vi "ChoosePass.vi"(8 "error in (no error)":errorcluster, 10 "Game":refnum<class "Game.lvclass">, 11 "Play in":refnum<class "Play.lvclass">) -> (0 "error out":errorcluster, 2 "Receptor passe":enum16{"Striker", "2nd Striker"}(ring), 3 "Play out":refnum<class "Play.lvclass">)   [LabVIEW 2018, in "Play.lvclass"]
uses:
  Play.lvclass
  Game_class/Game.lvclass
  Utilities_class/Utilities.lvclass
  Game_class/Game.lvclass/Game.ctl
  Team_class/Team.lvclass/Team.ctl
  Object_class/Object.lvclass/Object.ctl
  Robot_class/Robot.lvclass/Robot.ctl
  Referee_class/Referee.lvclass/Referee.ctl
  Object_class/Read x.vi
  Object_class/Read y.vi
  Robot_class/Read id.vi
  Referee_class/Read enemy_goalie_id.vi
  Team_class/Read RobotRef.vi
  Game_class/Read AllyRef.vi
  Game_class/Read BallRef.vi
  Game_class/Read FieldRef.vi
  Game_class/Read EnemyRef.vi
  Game_class/Read Referee.vi
  Ball_class/Ball.lvclass
  Ally_class/Ally.lvclass
  Robot_class/Robot.lvclass
  Enemy_class/Enemy.lvclass
  Field_class/Field.lvclass
  Referee_class/Referee.lvclass
panel:
  in  "x2":dbl=0.07
  in  "x1":dbl=0.16 format="%#_13g"
  in  "y 3":dbl=0.4 format="%#_13g"
  in  "y 2":dbl=0.17 format="%#_13g"
  in  "y":dbl=0.2 format="%#_13g"
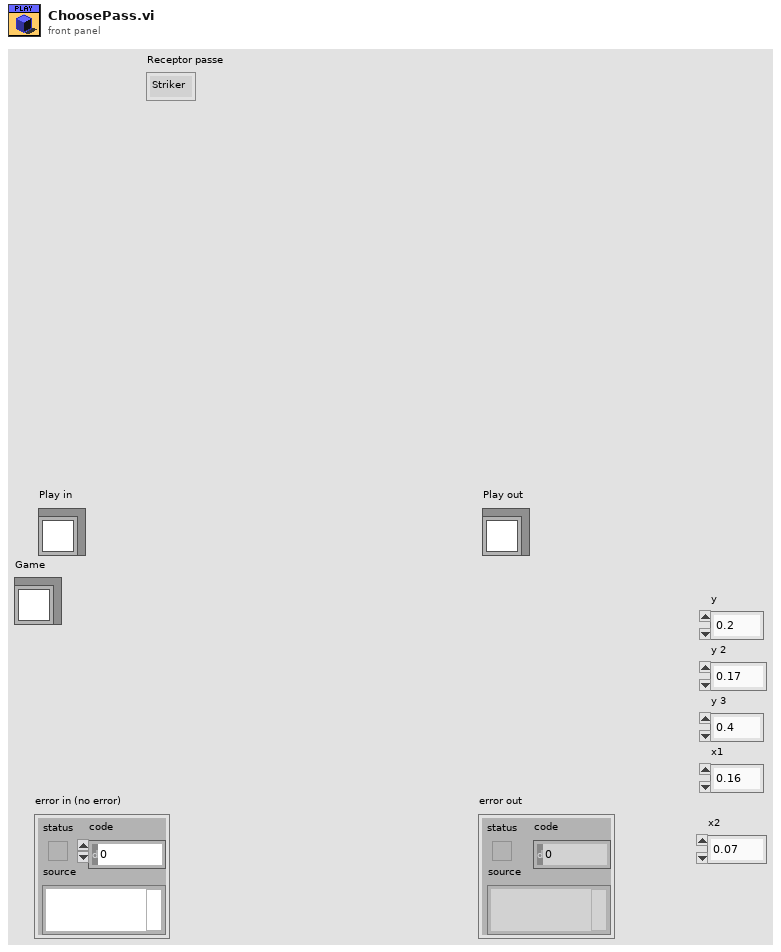
[diagram p1: front panel]
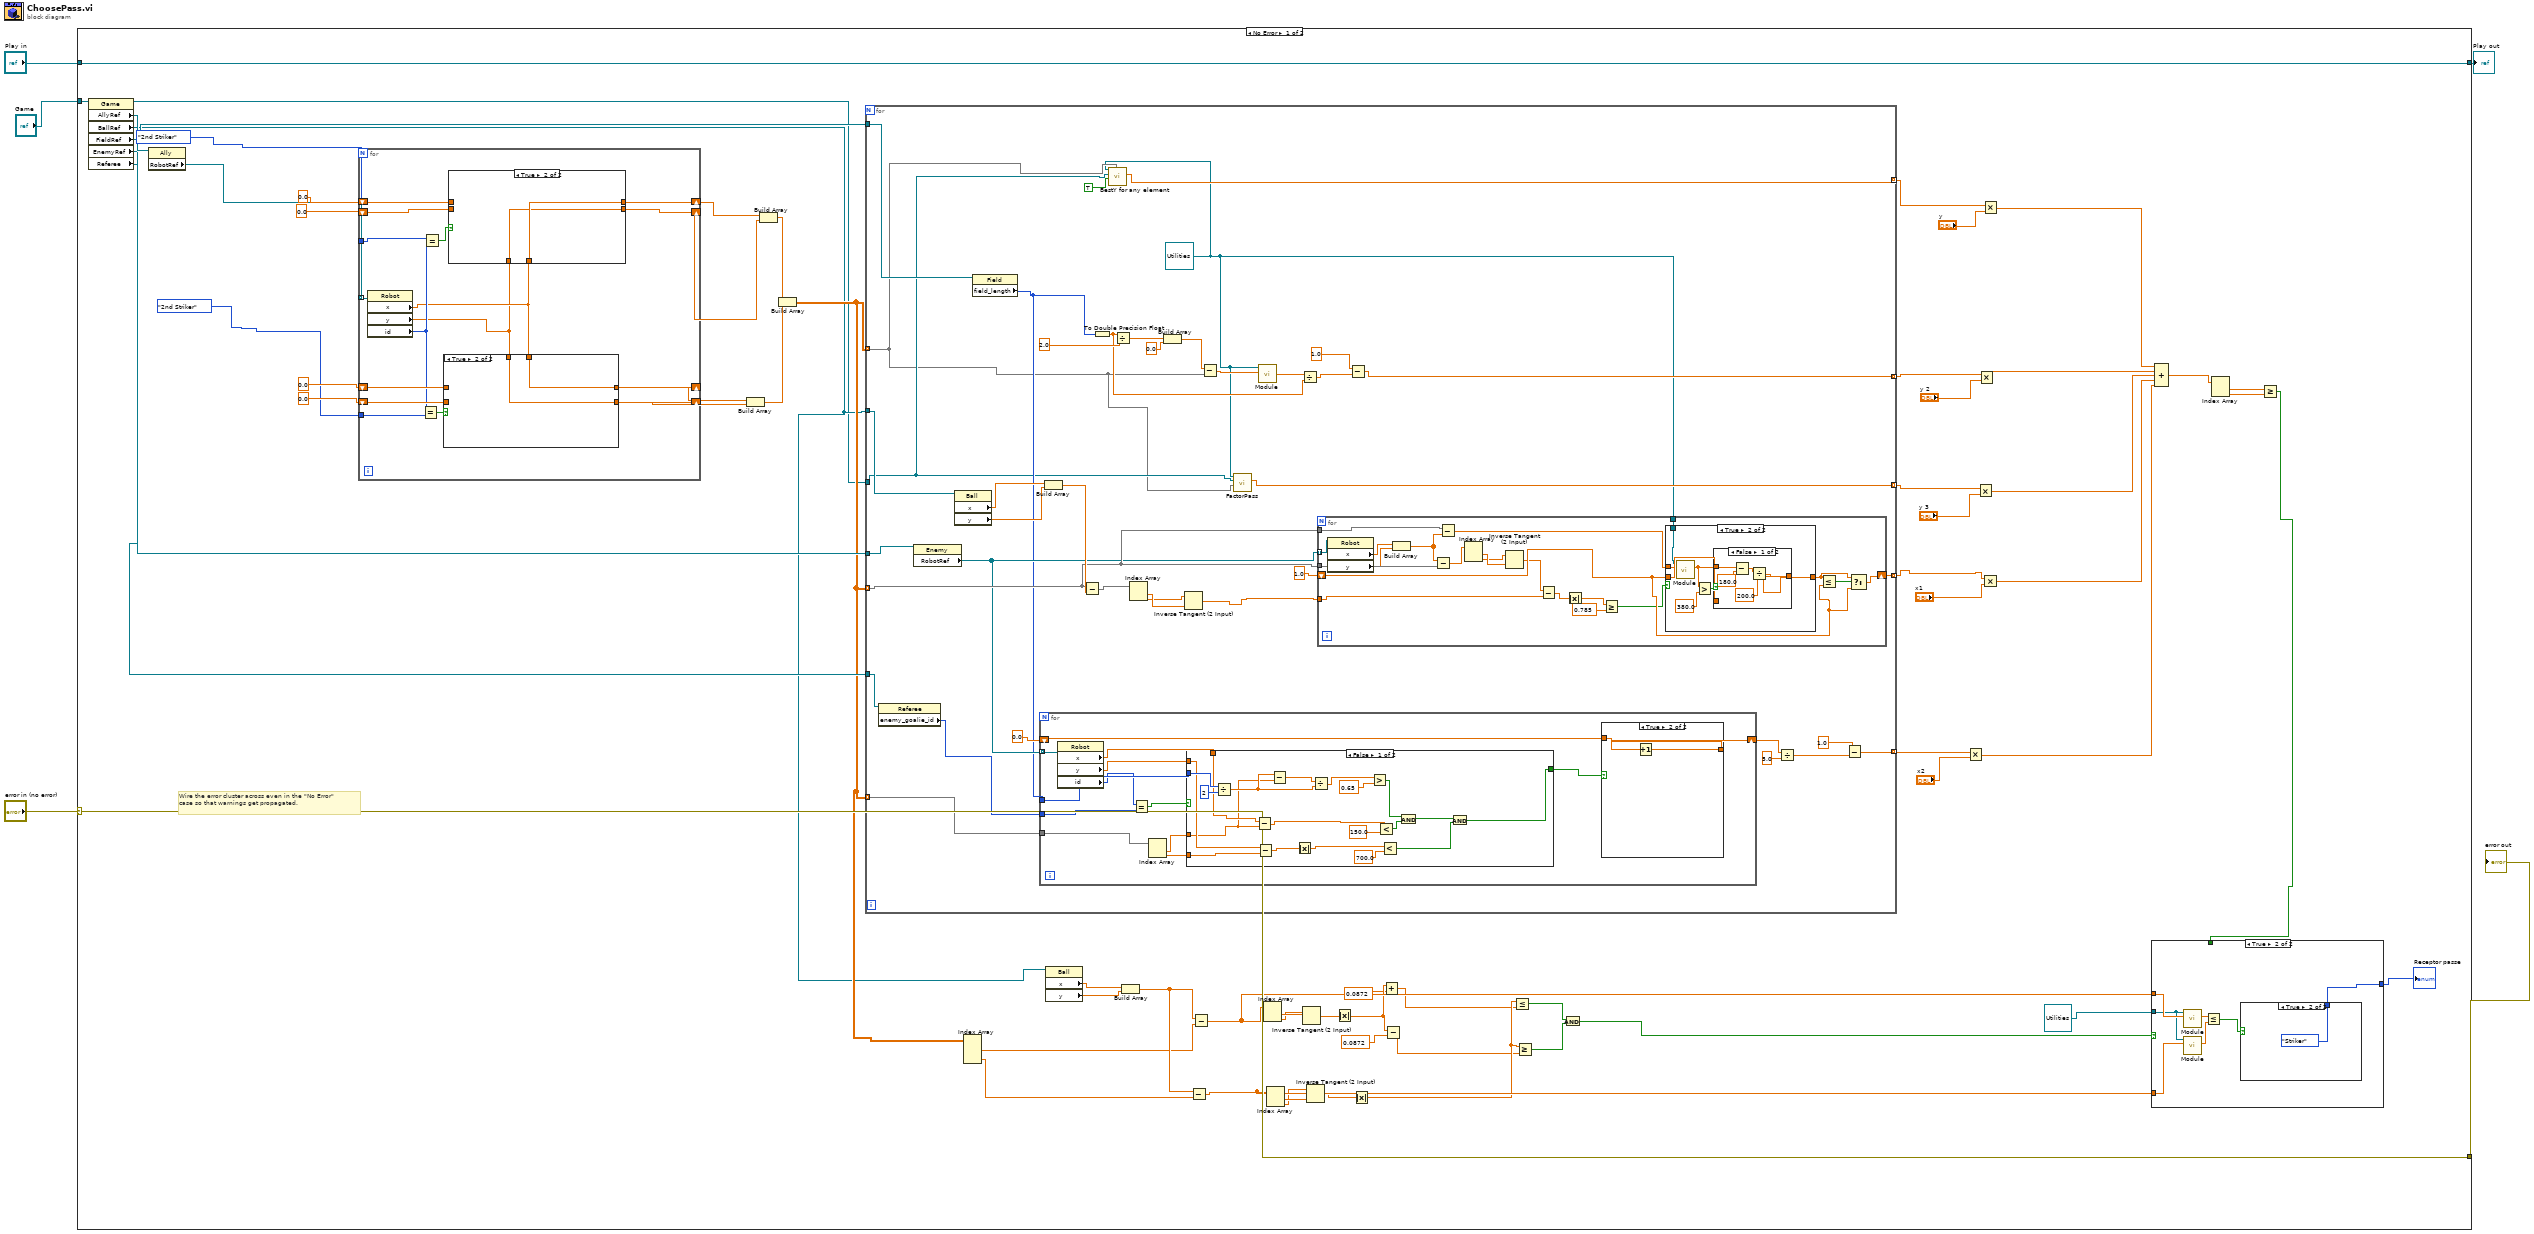
[diagram p0: block diagram]
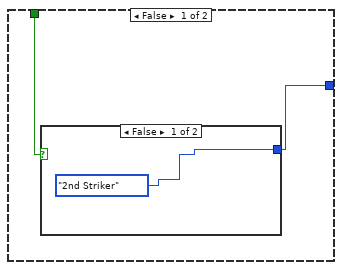
[diagram p2: hidden frame]
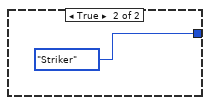
[diagram p3: hidden frame]
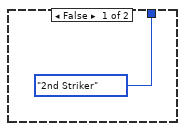
[diagram p4: hidden frame]
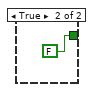
[diagram p5: hidden frame]
diagram:
  n1 = case shown="No Error" "error in (no error)" {
    selector: "error in (no error)" -> [w70 w222]
    tunnel: [w70 w222] -> w4
    tunnel: [w71 w221] -> w2
    tunnel: "Play in" -> [w71 w221]
    tunnel: "Game" -> [w69 _]
    frame No Error {
      # "Wire the error cluster across even in the \"No Error\"\ncase so that warnings get propagated."
      n2 = property class="Game"(reference=w69) -> (reference out=w7:refnum<class "Game.lvclass">, "AllyRef"=w68:refnum<class "Ally.lvclass">, "BallRef"=w31:refnum<class "Ball.lvclass">, "FieldRef"=w55:refnum<class "Field.lvclass">, "EnemyRef"=w54:refnum<class "Enemy.lvclass">, "Referee"=w53:refnum<class "Referee.lvclass">)  [unwired: 1 in, 1 out]
      n3 = property class="Ally"(reference=w68) -> ("RobotRef"=w57:refnum<class "Robot.lvclass">[])  [unwired: 1 in, 2 out]
      n4 = for {
        tunnel: w57 -> [w200] mode=indexing
        tunnel: enum16{"Striker", "2nd Striker"}."2nd Striker" ("Receptor passe") -> [w211]
        tunnel: enum16{"Striker", "2nd Striker"}."2nd Striker" ("Receptor passe") -> [w201]
        shift-right: [w210] -> w65
        shift-left: 0.0 ("x") -> [w209]
        shift-right: [w208] -> w64
        shift-left: 0.0 ("y") -> [w207]
        shift-right: [w205] -> w60
        shift-left: 0.0 ("y") -> [w203]
        shift-right: [w206] -> w61
        shift-left: 0.0 ("x") -> [w204]
        n5 = property class="Robot"(reference=w200) -> ("x"=w198:dbl, "y"=w197:dbl, "id"=w199:i32)  [unwired: 1 in, 2 out]
        n6 = Equal?(x=w199, y=w201) -> (x = y?=w202:bool)
        n7 = Equal?(x=w211, y=w199) -> (x = y?=w212:bool)
        n8 = case shown="True" w202 {
          tunnel: w198 -> [_ w216]
          tunnel: w197 -> [_ w215]
          tunnel: [w214 w216] -> w210
          tunnel: w209 -> [w214 _]
          tunnel: [w213 w215] -> w208
          tunnel: w207 -> [w213 _]
          frame False {
          }
          frame True {
          }
        }
        n9 = case shown="True" w212 {
          tunnel: w198 -> [_ w220]
          tunnel: w197 -> [_ w219]
          tunnel: [w218 w220] -> w206
          tunnel: [w217 w219] -> w205
          tunnel: w204 -> [w218 _]
          tunnel: w203 -> [w217 _]
          frame False {
          }
          frame True {
          }
        }
      }
      n10 = Build Array(w65, w64) -> (w66:dbl[])
      n11 = Build Array(w61, w60) -> (w67:dbl[])
      n12 = Build Array(w67, w66) -> (w32:dbl[][])
      n13 = for {
        tunnel: w32 -> [w86] mode=indexing
        tunnel: [w89] -> w10 mode=indexing
        tunnel: [w117] -> w11 mode=indexing
        tunnel: [w90] -> w12 mode=indexing
        tunnel: w32 -> [w111] mode=indexing
        tunnel: [w114] -> w13 mode=indexing
        tunnel: w32 -> [w108] mode=indexing
        tunnel: [w102] -> w14 mode=indexing
        tunnel: w31 -> [w101]
        tunnel: w55 -> [w91]
        tunnel: w54 -> [w96]
        tunnel: w53 -> [w93]
        tunnel: w7 -> [w87]
        w85 = refnum<class "Utilities.lvclass"> refnum ("Utilities in")
        n14 = property class="Referee"(reference=w93) -> ("enemy_goalie_id"=w92:i32)  [unwired: 1 in, 2 out]
        n15 = property class="Enemy"(reference=w96) -> ("RobotRef"=w95:refnum<class "Robot.lvclass">[])  [unwired: 1 in, 2 out]
        n16 = property class="Ball"(reference=w101) -> ("x"=w100:dbl, "y"=w99:dbl)  [unwired: 1 in, 2 out]
        n17 = property class="Field"(reference=w91) -> ("field_length"=w94:i32)  [unwired: 1 in, 2 out]
        n18 = for {
          tunnel: w108 -> [w131]
          shift-right: [w136] -> w106
          shift-left: 0.0 ("x") -> [w137]
          tunnel: w92 -> [w135]
          tunnel: w94 -> [w132]
          tunnel: w95 -> [w128] mode=indexing
          n19 = property class="Robot"(reference=w128) -> ("x"=w127:dbl, "y"=w126:dbl, "id"=w125:i32)  [unwired: 1 in, 2 out]
          n20 = Equal?(x=w125, y=w135) -> (x = y?=w134:bool)
          n21 = Index Array(array=w131) -> (element #1=w130:dbl, element #2=w129:dbl)  [unwired: 2 in]
          n22 = case shown="False" w134 {
            tunnel: [w139 FALSE] -> w133
            tunnel: w132 -> [w157 _]
            tunnel: w127 -> [w150 _]
            tunnel: w130 -> [w138 _]
            tunnel: w126 -> [w148 _]
            tunnel: w129 -> [w147 _]
            frame False {
              n23 = Divide(x=w157, y=u32 2) -> (x/y=w154:dbl)
              n24 = Subtract(x=w150, y=w138) -> (x-y=w149:dbl)
              n25 = Subtract(x=w148, y=w147) -> (x-y=w146:dbl)
              n26 = Subtract(x=w154, y=w138) -> (x-y=w155:dbl)
              n27 = Absolute Value(x=w146) -> (abs(x)=w145:dbl)
              n28 = Divide(x=w155, y=w154) -> (x/y=w153:dbl)
              n29 = Greater?(x=w153, y=0.65) -> (0:w143:bool)
              n30 = Less?(x=w149, y=150.0) -> (x < y?=w142:bool)
              n31 = Less?(x=w145, y=700.0) -> (x < y?=w140:bool)
              n32 = And(x=w143, y=w142) -> (x .and. y?=w141:bool)
              n33 = And(x=w141, y=w140) -> (x .and. y?=w139:bool)
            }
            frame True {
            }
          }
          n34 = case shown="True" w133 {
            tunnel: w137 -> [w159 w161]
            tunnel: [w159 w160] -> w136
            frame False {
            }
            frame True {
              n35 = Increment(x=w161) -> (x+1=w160:dbl)
            }
          }
        }
        n36 = Build Array(w100, w99) -> (w113:dbl[])
        n37 = Subtract(x=w111, y=w113) -> (x-y=w116:dbl[])
        n38 = To Double Precision Float(number=w94) -> (double precision float=w120:dbl)
        n39 = call-dynamic "BestY for any element.vi"("Element Position"=w86, "Enemys(T)\nAllys(F)"=TRUE ("Maior intervalo(T)\nMaior angulo(F)"), "Game"=w87, "Utilities in"=w85) -> ("Goal Gap Normalizado(%do gol aberta)"=w89:dbl)  [unwired: 5 in, 2 out]
        n40 = Divide(x=w120, y=2.0) -> (x/y=w123:dbl)
        n41 = Index Array(array=w116) -> (element #1=w110:dbl, element #2=w109:dbl)  [unwired: 2 in]
        n42 = Build Array(w123, 0.0 ("element")) -> (w122:dbl[])
        n43 = Inverse Tangent (2 Input)(1:w110, 2:w109) -> (0:w112:dbl)
        n44 = Subtract(x=w122, y=w86) -> (x-y=w97:dbl[])
        n45 = call-dynamic "FactorPass.vi"("Coordenada robo"=w86, "Game"=w87, "Utilities in"=w85) -> ("Critério de marcação Normalizado"=w90:dbl)  [unwired: 6 in, 2 out]
        n46 = call-dynamic "Module.vi"("2D vector"=w97, "Utilities in"=w85) -> ("Modulo"=w98:dbl)  [unwired: 7 in, 2 out]
        n47 = Divide(x=w98, y=w120) -> (x/y=w118:dbl)
        n48 = for {
          tunnel: w112 -> [w173]
          tunnel: w111 -> [w181]
          shift-right: [w175] -> w114
          shift-left: 1.0 ("x") -> [w176]
          tunnel: w111 -> [w179]
          tunnel: w95 -> [w165] mode=indexing
          tunnel: w85 -> [w162]
          n49 = property class="Robot"(reference=w165) -> ("x"=w164:dbl, "y"=w163:dbl)  [unwired: 1 in, 2 out]
          n50 = Build Array(w164, w163) -> (w180:dbl[])
          n51 = Subtract(x=w180, y=w181) -> (x-y=w182:dbl[])
          n52 = Subtract(x=w179, y=w180) -> (x-y=w178:dbl[])
          n53 = Index Array(array=w182) -> (element #1=w167:dbl, element #2=w166:dbl)  [unwired: 2 in]
          n54 = Inverse Tangent (2 Input)(1:w167, 2:w166) -> (0:w172:dbl)
          n55 = Subtract(x=w172, y=w173) -> (x-y=w171:dbl)
          n56 = Absolute Value(x=w171) -> (abs(x)=w170:dbl)
          n57 = Greater Or Equal?(x=w170, y=0.785) -> (x >= y?=w169:bool)
          n58 = case shown="True" w169 {
            tunnel: w178 -> [_ w186]
            tunnel: w176 -> [w183 w188]
            tunnel: [w183 w187] -> w177
            tunnel: w162 -> [_ w184]
            frame False {
            }
            frame True {
              n59 = call-dynamic "Module.vi"("2D vector"=w186, "Utilities in"=w184) -> ("Modulo"=w185:dbl)  [unwired: 7 in, 2 out]
              n60 = Greater?(x=w185, y=380.0) -> (0:w189:bool)
              n61 = case shown="False" w189 {
                tunnel: w188 -> [_ w196]
                tunnel: [w195 w196] -> w187
                tunnel: w185 -> [w194 _]
                frame False {
                  n62 = Subtract(x=w194, y=180.0) -> (x-y=w192:dbl)
                  n63 = Divide(x=w192, y=200.0) -> (x/y=w195:dbl)
                }
                frame True {
                }
              }
            }
          }
          n64 = Less Or Equal?(x=w177, y=w176) -> (x <= y?=w174:bool)
          n65 = Select(t=w177, s=w174, f=w176) -> (s? t:f=w175:dbl)
        }
        n66 = Subtract(x=1.0, y=w118) -> (x-y=w117:dbl)
        n67 = Divide(x=w106, y=5.0) -> (x/y=w104:dbl)
        n68 = Subtract(x=1.0 ("y"), y=w104) -> (x-y=w102:dbl)
      }
      n69 = Index Array(array=w32) -> (element #1=w34:dbl[], element #2=w33:dbl[])  [unwired: 4 in]
      n70 = property class="Ball"(reference=w31) -> ("x"=w30:dbl, "y"=w29:dbl)  [unwired: 1 in, 2 out]
      n71 = Build Array(w30, w29) -> (w50:dbl[])
      n72 = Subtract(x=w50, y=w33) -> (x-y=w51:dbl[])
      n73 = Subtract(x=w50, y=w34) -> (x-y=w52:dbl[])
      n74 = Index Array(array=w52) -> (element #1=w36:dbl, element #2=w35:dbl)  [unwired: 2 in]
      n75 = Index Array(array=w51) -> (element #1=w40:dbl, element #2=w39:dbl)  [unwired: 2 in]
      n76 = Inverse Tangent (2 Input)(1:w36, 2:w35) -> (0:w41:dbl)
      n77 = Inverse Tangent (2 Input)(1:w40, 2:w39) -> (0:w43:dbl)
      n78 = Absolute Value(x=w41) -> (abs(x)=w42:dbl)
      n79 = Absolute Value(x=w43) -> (abs(x)=w46:dbl)
      n80 = Add(x=w42, y=0.0872) -> (x+y=w44:dbl)
      n81 = Subtract(x=w42, y=0.0872) -> (x-y=w45:dbl)
      n82 = Less Or Equal?(x=w46, y=w44) -> (x <= y?=w47:bool)
      n83 = Greater Or Equal?(x=w46, y=w45) -> (x >= y?=w48:bool)
      n84 = And(x=w47, y=w48) -> (x .and. y?=w49:bool)
      n85 = Multiply(x=w14, y="x2") -> (x*y=w17:dbl[])
      n86 = Multiply(x=w12, y="y 3") -> (x*y=w23:dbl[])
      n87 = Multiply(x=w11, y="y 2") -> (x*y=w24:dbl[])
      n88 = Multiply(x=w13, y="x1") -> (x*y=w18:dbl[])
      n89 = Multiply(x=w10, y="y") -> (x*y=w25:dbl[])
      n90 = Compound Arithmetic op=ADD(w25, w24, w23, w18, w17) -> (w22:dbl[])
      n91 = Index Array(array=w22) -> (element #1=w21:dbl, element #2=w20:dbl)  [unwired: 2 in]
      n92 = Greater Or Equal?(x=w21, y=w20) -> (x >= y?=w15:bool)
      n93 = case shown="True" w49 {
        tunnel: w51 -> [_ w80]
        tunnel: w52 -> [_ w77]
        tunnel: w15 -> [w73 _]
        tunnel: [w72 w81] -> w6
        tunnel: refnum<class "Utilities.lvclass"> refnum ("Utilities in") -> [_ w76]
        frame False {
          n94 = case shown="False" w73 {
            tunnel: [enum16{"Striker", "2nd Striker"}."2nd Striker" ("Receptor passe") enum16{"Striker", "2nd Striker"}."Striker" ("Receptor passe")] -> w72
            frame False {
            }
            frame True {
            }
          }
        }
        frame True {
          n95 = call-dynamic "Module.vi"("2D vector"=w77, "Utilities in"=w76) -> ("Modulo"=w78:dbl)  [unwired: 7 in, 2 out]
          n96 = call-dynamic "Module.vi"("2D vector"=w80, "Utilities in"=w76) -> ("Modulo"=w79:dbl)  [unwired: 7 in, 2 out]
          n97 = Less Or Equal?(x=w78, y=w79) -> (x <= y?=w82:bool)
          n98 = case shown="True" w82 {
            tunnel: [enum16{"Striker", "2nd Striker"}."2nd Striker" ("Receptor passe") enum16{"Striker", "2nd Striker"}."Striker" ("Receptor passe")] -> w81
            frame False {
            }
            frame True {
            }
          }
        }
      }
      "Receptor passe" <- w6
    }
    frame Error {
    }
  }
  "error out" <- w4
  "Play out" <- w2
